vi "Hardware-HHScope.vi"(11 "DSI Reference":refnum<class "DCM-DSI.lvclass">) -> ()   [LabVIEW 2016, in "DSI-RT.lvlib"]
uses:
  DSI-RT.lvlib
  Classes/DCM-DSI/DCM-DSI.lvclass
  <vilib>/Powertrain Controls/Device Drivers/DCM/Rev0/RT/DCM - RT.lvclass/DCM - RT.ctl
  <vilib>/Powertrain Controls/Device Drivers/DCM/Rev0/RT/Read Stop Target.vi
  Classes/DCM-DSI/Read DCM Ref.vi
  Classes/DCM-DSI/Write HH Scope Data.vi
  <vilib>/Powertrain Controls/Device Drivers/DCM/Rev0/RT/DCM - RT.lvclass
  <vilib>/addons/Software Calibration Management/xSCM/CalPoint.xnode
  <vilib>/Powertrain Controls/Device Drivers/DCM/HH/RT/DCM - RT - HH.lvlib
  <vilib>/addons/Software Calibration Management/xSCM/ni_scm.dll
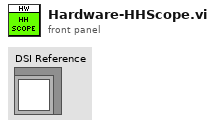
[diagram p1: front panel]
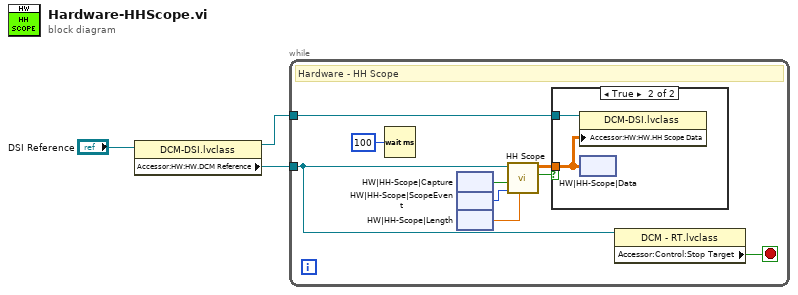
[diagram p0: block diagram]
diagram:
  n1 = property class="DCM-DSI.lvclass"(reference="DSI Reference") -> (reference out=w1:refnum<class "DCM-DSI.lvclass">, "Accessor:HW:HW.DCM Reference"=w2:refnum<class "DCM - RT.lvclass">)  [unwired: 1 in, 1 out]
  n2 = while {
    tunnel: w2 -> [w7]
    tunnel: w1 -> [w6]
    stop <- w8 stop-if-true
    # "Hardware - HH Scope"
    n3 = Wait (ms)(milliseconds to wait=u32 100) -> ()  [unwired: 1 out]
    n4 = xnode "HW|HH-Scope|Capture"() -> ("Value"=w9:bool)
    n5 = xnode "HW|HH-Scope|ScopeEvent"() -> ("Value"=w4:u8)
    n6 = xnode "HW|HH-Scope|Length"() -> ("Value"=w5:sgl)
    n7 = call <vilib>:"HH Scope.vi"("HH Scope Length [s]"=w5, "HH Scope Event"=w4, "HH Scope Capture"=w9, "DCM Reference"=w7) -> ("New Data"=w12:bool, "Data"=w11:sgl[][])  [unwired: 4 in, 2 out]
    n8 = case shown="True" w12 {
      tunnel: w11 -> [_ w28]
      tunnel: w6 -> [_ w29]
      frame False {
      }
      frame True {
        n9 = property class="DCM-DSI.lvclass"(reference=w29, "Accessor:HW:HW.HH Scope Data"=w28) -> ()  [unwired: 1 in, 2 out]
        n10 = xnode "HW|HH-Scope|Data"("Value"=w28) -> ()
      }
    }
    n11 = property class="DCM - RT.lvclass"(reference=w7) -> ("Accessor:Control:Stop Target"=w8:bool)  [unwired: 1 in, 2 out]
  }
